vi "Main.vi"(10 "JQMHStartup.lvclass":refnum<class "JQMHStartup.lvclass">, 11 "TesterModule in":refnum<class "TesterModule.lvclass">) -> ()   [LabVIEW 2024, in "TesterModule.lvclass"]
uses:
  TesterModule.lvclass
  C:/Github/JQMH/JQMHCore/Module/JQMHModule.lvclass
  JQMHCore/JQMHStartup/JQMHStartup.lvclass
  JQMHCore/Module/JQMHModule.lvclass/JQMHModule.ctl
  Message Queue_class/Delacor_lib_QMH_Message Queue.lvclass
  TesterModule.lvclass/TesterModule.ctl
  JQMHCore/Shared/JQMHShared.lvlib
  JQMHCore/Module/JQMHModule.lvclass
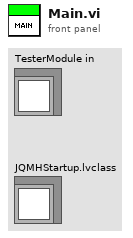
[diagram p1: front panel]
types:
  T1 = typedef "JQMHModule.lvclass/StandardEvents.ctl" = cluster{"Stop Module":refnum<user-event>}
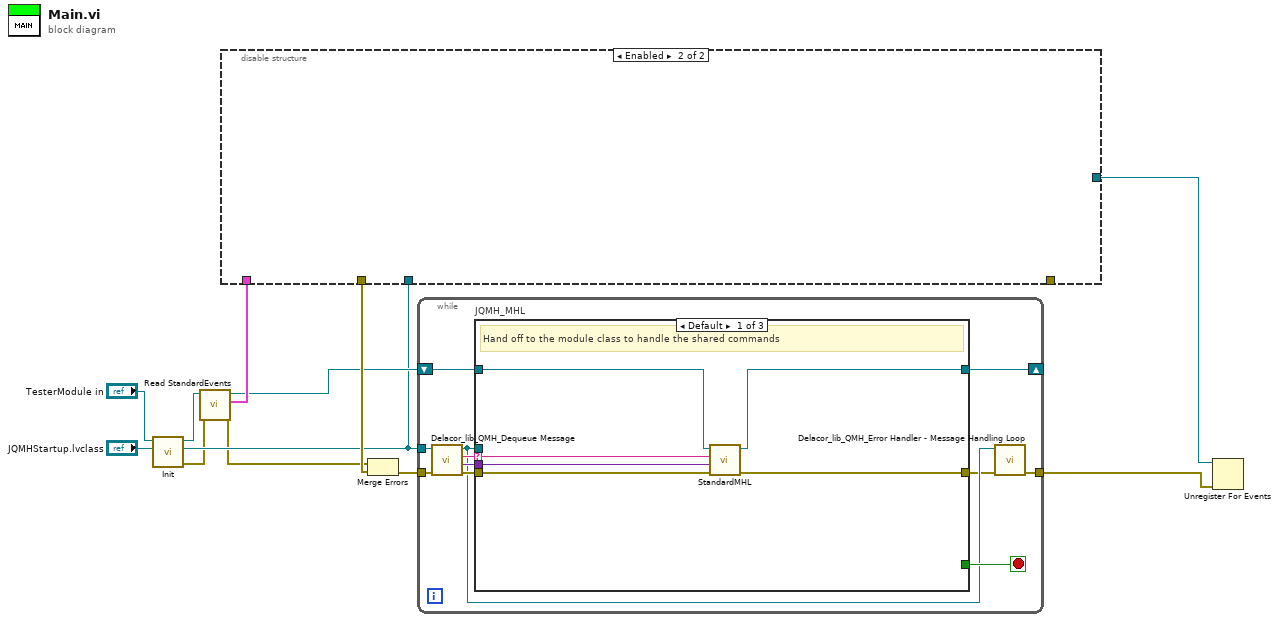
[diagram p0: block diagram]
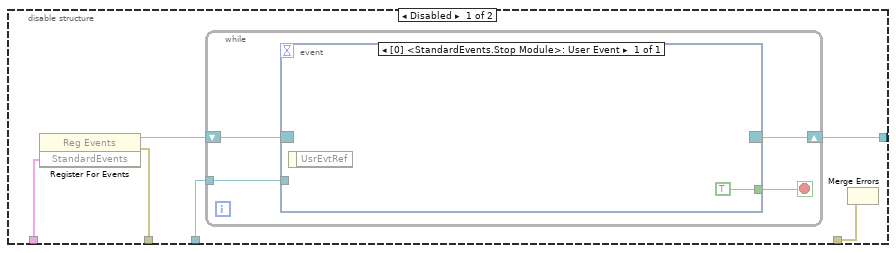
[diagram p2: hidden frame]
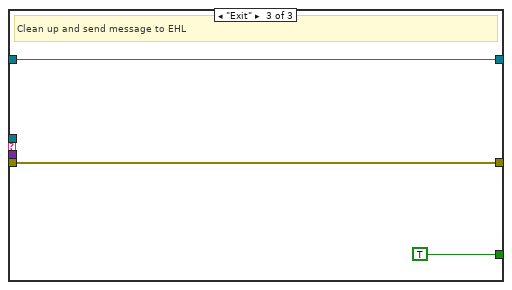
[diagram p4: hidden frame]
diagram:
  n1 = call "Init.vi"("JQMHStartup.lvclass"="JQMHStartup.lvclass", "JQMHCore.lvclass"="TesterModule in") -> ("error out"=w3:errorcluster, "Message Queue"=w7:refnum<class "Delacor_lib_QMH_Message Queue.lvclass">, "JQMHCore out"=w4:refnum<class "TesterModule.lvclass">)  [unwired: 6 in, 1 out]
  n2 = call "Read StandardEvents.vi"("error in (no error)"=w3, "JQMHCore in"=w4) -> ("error out"=w2:errorcluster, "StandardEvents"=w10:T1, "JQMHCore out"=w9:refnum<class "TesterModule.lvclass">)  [unwired: 7 in]
  n3 = disable-structure shown="Enabled" {
    disable-tunnel: [w18 _] -> w11
    disable-tunnel: w10 -> [w17 _]
    disable-tunnel: [w15 _] -> w8
    disable-tunnel: w7 -> [w14 _]
    disable-tunnel: _ -> [w13 _]
    frame Disabled {
      n4 = register-events(w17) -> (reference out=w16:refnum<event-registration>, error out=w18:errorcluster)  [unwired: 2 in]
      n5 = while {
        shift-right: [w21] -> w15
        shift-left: w16 -> [w22]
        tunnel: w14 -> [w19]
        stop <- w20 stop-if-true
        n6 = event shown="[0] <StandardEvents.Stop Module>: User Event" {
          selector: w22 -> [_]
          dyn-events: [_] -> w21
          timeout: _ -> [_]
          tunnel: [TRUE] -> w20
          tunnel: w19 -> [_]
          event User Event {
            n7 = event-data() -> ()  [unwired: 1 in, 1 out]
          }
        }
      }
      n8 = Merge Errors(w13) -> ()  [unwired: 1 in, 1 out]
    }
    frame Enabled {
    }
  }
  n9 = Merge Errors(w2, w11) -> (w12:errorcluster)
  n10 = while {
    tunnel: w7 -> [w34]
    tunnel: w12 -> [w32]
    shift-right: [w25] -> _
    shift-left: w9 -> [w30]
    tunnel: [w24] -> w1
    stop <- w31 stop-if-true
    n11 = call-dynamic "Delacor_lib_QMH_Dequeue Message.vi"("error in"=w32, "Message Queue in"=w34) -> ("error out"=w28:errorcluster, "Message Data"=w29:variant, "Message"=w33:string, "Message Queue out"=w27:refnum<class "Delacor_lib_QMH_Message Queue.lvclass">)  [unwired: 6 in]
    n12 = case "JQMH_MHL" shown="Default" w33 {
      selector: w33 -> [w37 _ _]
      tunnel: [_ _ TRUE] -> w31
      tunnel: w30 -> [w38 w42 w43]
      tunnel: w29 -> [w36 _ _]
      tunnel: w28 -> [w39 w41 w44]
      tunnel: w27 -> [_ _ _]
      tunnel: [w40 w41 w44] -> w26
      tunnel: [w35 w42 w43] -> w25
      frame Default {
        # "Hand off to the module class to handle the shared commands"
        n13 = call-dynamic "StandardMHL.vi"("error in (no error)"=w39, "Message Data"=w36, "Message"=w37, "JQMHModule in"=w38) -> ("error out"=w40:errorcluster, "JQMHModule out"=w35:refnum<class "TesterModule.lvclass">)  [unwired: 6 in]
      }
      frame "Initalise" {
      }
      frame "Exit" {
        # "Clean up and send message to EHL"
      }
    }
    n14 = call-dynamic "Delacor_lib_QMH_Error Handler - Message Handling Loop.vi"("error in"=w26, "Message Queue in"=w27) -> ("dup error in"=w24:errorcluster)  [unwired: 8 in, 1 out]
  }
  n15 = Unregister For Events(event registration refnum=w8, error in=w1) -> ()  [unwired: 1 out]
